vi "PH_SSAC.create i Attrib.vi"() -> (0 "i Attr":T1={"GUI Refs"={"Delete"=refnum, "Global On"=refnum, "Cam Source"=refnum, "Frame Main Signal"=refnum, "Frame Background"=refnum, "dt (Gauss smooth)"=refnum, "Calibration Factor"=refnum, "Background acquire"=refnum, "Threshold"=refnum, "Time evolution of mean pulse duration"=refnum, "Mean Pulse Duration"=refnum, "Main signal"=refnum, "Current Pulse Duration"=refnum, "Processed"=refnum, "Saturation"=refnum, "# for Average"=refnum, "Position"=refnum, "BG Status"=refnum, "Save BG data"=refnum, "Read BG Data"=refnum, "Background Calibration Data"=refnum}, "Images"={"OP Image"=refnum, "GUI Image"=refnum, "PSDB Image"=refnum}, "Global On?"=FALSE, "Frame Main"={"x"=0, "dx"=1280, "y"=150, "dy"=150}, "Frame Background"={"x"=0, "dx"=100, "y"=400, "dy"=250}, "dt [fs]"=1.0, "Calibration Factor [fs/pixel]"=1.0, "Threshold"=0.0, "Time evolution of mean pulse duration [fs]"=[], "Main Signal"={"Time for Main"=[], "Signal"=[]}, "Processed"=FALSE, "Current Pulse Duration [fs]"=0.0, "# for Average"=1, "Position"=0, "Pulse Durations [fs]"=[], "BG"={"Acquire?"=FALSE, "Background Calibration Data"={"Date"="", "Time"="", "Frame Main"={"x"=0, "dx"=0, "y"=0, "dy"=0}, "dt [fs]"=0.0, "Calibration Factor [fs/pixel]"=0.0, "Signal"=array[1280 elements], "Frame Background"={"x"=0, "dx"=100, "y"=400, "dy"=250}}, "Save Data"=FALSE}})   [LabVIEW 2014, in "PH_SSAC.lvlib"]
doc: "In this VI the related instances which are not set in the Read DB Vi are defined and set to own attributes."
uses:
  PH_SSAC.lvlib
  PH_SSAC.i attribute.ctl
  <vilib>/vision/Image Controls.llb/IMAQ Image.ctl
  PH_SSAC.Background Data.ctl
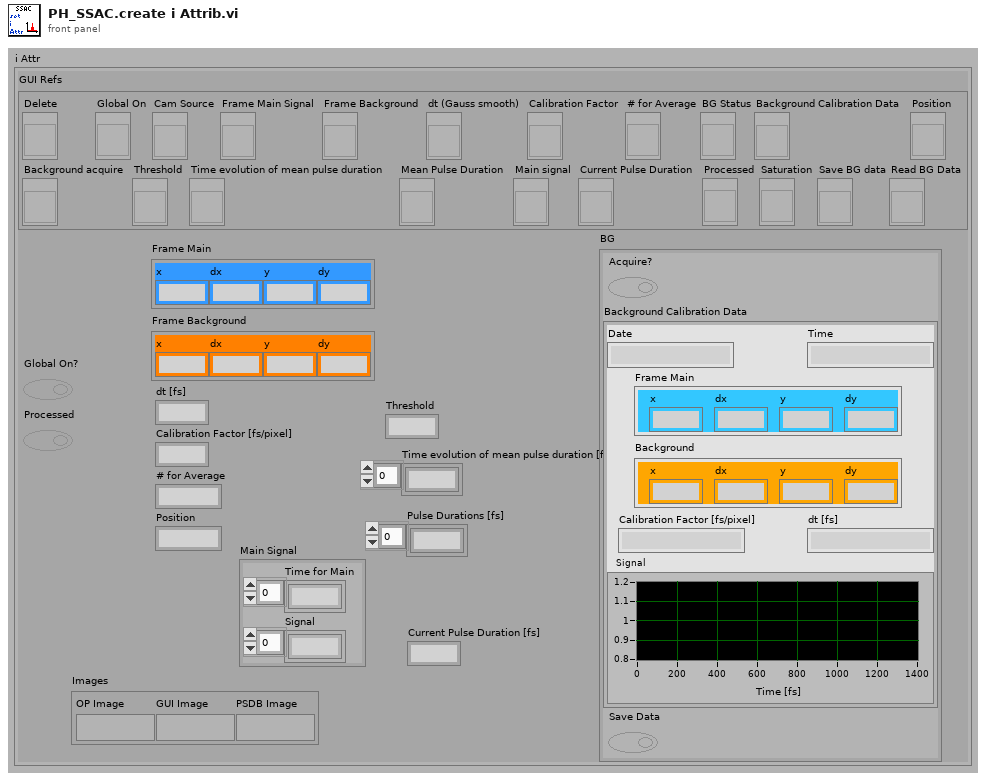
[diagram p1: front panel]
types:
  T1 = typedef "PH_SSAC.lvlib/PH_SSAC.i attribute.ctl" = cluster{"GUI Refs":cluster{"Delete":refnum<vi>, "Global On":refnum<vi>, "Cam Source":refnum<vi>, "Frame Main Signal":refnum<vi>, "Frame Background":refnum<vi>, "dt (Gauss smooth)":refnum<vi>, "Calibration Factor":refnum<vi>, "Background acquire":refnum<vi>, "Threshold":refnum<vi>, "Time evolution of mean pulse duration":refnum<vi>, "Mean Pulse Duration":refnum<vi>, "Main signal":refnum<vi>, "Current Pulse Duration":refnum<vi>, "Processed":refnum<vi>, "Saturation":refnum<vi>, "# for Average":refnum<vi>, "Position":refnum<vi>, "BG Status":refnum<vi>, "Save BG data":refnum<vi>, "Read BG Data":refnum<vi>, "Background Calibration Data":refnum<vi>}, "Images":cluster{"OP Image":T2, "GUI Image":T2, "PSDB Image":T2}, "Global On?":bool, "Frame Main":cluster{"x":u32, "dx":u32, "y":u32, "dy":u32}, "Frame Background":cluster{"x":u32, "dx":u32, "y":u32, "dy":u32}, "dt [fs]":dbl, "Calibration Factor [fs/pixel]":dbl, "Threshold":dbl, "Time evolution of mean pulse duration [fs]":dbl[], "Main Signal":cluster{"Time for Main":dbl[], "Signal":dbl[]}, "Processed":bool, "Current Pulse Duration [fs]":dbl, "# for Average":i32, "Position":i32, "Pulse Durations [fs]":dbl[], "BG":cluster{"Acquire?":bool, "Background Calibration Data":T3, "Save Data":bool}}
  T2 = typedef "IMAQ Image.ctl" = refnum<image>
  T3 = typedef "PH_SSAC.lvlib/PH_SSAC.Background Data.ctl" = cluster{"Date":string, "Time":string, "Frame Main":cluster{"x":u32, "dx":u32, "y":u32, "dy":u32}, "dt [fs]":dbl, "Calibration Factor [fs/pixel]":dbl, "Signal":dbl[], "Frame Background":cluster{"x":u32, "dx":u32, "y":u32, "dy":u32}}
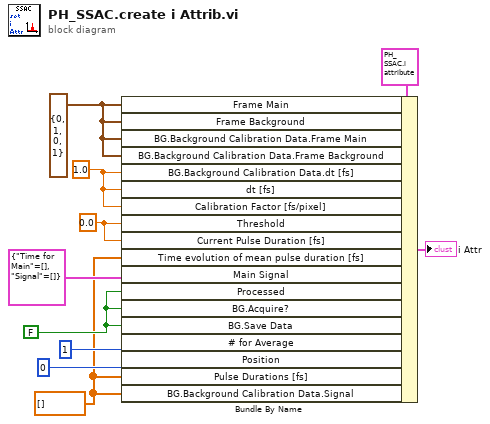
[diagram p0: block diagram]
diagram:
  w3 = dbl[] [] ("Pulse Durations [fs]")
  w4 = FALSE ("Processed")
  w5 = 0.0 ("Threshold")
  w6 = 1.0 ("dt [fs]")
  w7 = cluster{"x":u32, "dx":u32, "y":u32, "dy":u32} {"x"=0, "dx"=1, "y"=0, "dy"=1} ("Frame Main")
  n1 = Bundle By Name(cluster=T1 {"GUI Refs"={"Delete"=refnum, "Global On"=refnum, "Cam Source"=refnum, "Frame Main Signal"=refnum, "Frame Background"=refnum, "dt (Gauss smooth)"=refnum, "Calibration Factor"=refnum, "Background acquire"=refnum, "Threshold"=refnum, "Time evolution of mean pulse duration"=refnum, "Mean Pulse Duration"=refnum, "Main signal"=refnum, "Current Pulse Duration"=refnum, "Processed"=refnum, "Saturation"=refnum, "# for Average"=refnum, "Position"=refnum, "BG Status"=refnum, "Save BG data"=refnum, "Read BG Data"=refnum, "Background Calibration Data"=refnum}, "Images"={"OP Image"=refnum, "GUI Image"=refnum, "PSDB Image"=refnum}, "Global On?"=FALSE, "Frame Main"={"x"=0, "dx"=0, "y"=0, "dy"=0}, "Frame Background"={"x"=0, "dx"=0, "y"=0, "dy"=0}, "dt [fs]"=0.0, "Calibration Factor [fs/pixel]"=0.0, "Threshold"=0.0, "Time evolution of mean pulse duration [fs]"=[], "Main Signal"={"Time for Main"=[], "Signal"=[]}, "Processed"=FALSE, "Current Pulse Duration [fs]"=0.0, "# for Average"=0, "Position"=0, "Pulse Durations [fs]"=[], "BG"={"Acquire?"=FALSE, "Background Calibration Data"={"Date"="", "Time"="", "Frame Main"={"x"=0, "dx"=0, "y"=0, "dy"=0}, "dt [fs]"=0.0, "Calibration Factor [fs/pixel]"=0.0, "Signal"=[], "Frame Background"={"x"=0, "dx"=0, "y"=0, "dy"=0}}, "Save Data"=FALSE}} ("i Attr"), "Frame Main"=w7, "Frame Background"=w7, "BG.Background Calibration Data.Frame Main"=w7, "BG.Background Calibration Data.Frame Background"=w7, "BG.Background Calibration Data.dt [fs]"=w6, "dt [fs]"=w6, "Calibration Factor [fs/pixel]"=w6, "Threshold"=w5, "Current Pulse Duration [fs]"=w5, "Time evolution of mean pulse duration [fs]"=w3, "Main Signal"=cluster{"Time for Main":dbl[], "Signal":dbl[]} {"Time for Main"=[], "Signal"=[]}, "Processed"=w4, "BG.Acquire?"=w4, "BG.Save Data"=w4, "# for Average"=1, "Position"=0, "Pulse Durations [fs]"=w3, "BG.Background Calibration Data.Signal"=w3) -> (→"i Attr":T1)
